vi "Pfeiffer-RVC300.close interface.vi"(0 "i ref in":refnum<vi>, 3 "ms timeout (10000)":i32=10000, 5 "error in (no error)":errorcluster) -> (14 "i ref out":refnum<vi>, 17 "timed out":bool, 19 "error out":errorcluster)   [LabVIEW 2014, in "Pfeiffer-RVC300.lvlib"]
doc: "Closes the interface to the instrument.\n\nLicense Agreement for this software:\n\nCopyright (C)\nMax-Planck-Institut für Kernphysik\nSaupfercheckweg 1\n69117 Heidelberg\nGermany\n\nContact: christopher.borgmann@mpi-hd.mpg.de\n\nThis program is free software: you can redistribute it and/or modify \nit under the terms of the GNU General Public License as published by\nthe Free Software Foundation, either version 3 of the License, or\n(at your option) any later version.\n\nThis program is distributed in the hope that it will be useful,\nbut WITHOUT ANY WARRANTY; without even the implied warranty of\nMERCHANTABILITY or FITNESS FOR A PARTICULAR PURPOSE. See the\nGNU General Public License for more details.\n\nYou should have received a copy of the GNU General Public License\nalong with this program. If not, see <http://www.gnu.org/licenses/>.\n\nMax-Planck-Institut für Kernphysik\nSaupfercheckweg 1, 69117 Heidelberg, Germany\nFor all questions and ideas contact: christopher.borgmann@mpi-hd.mpg.de\nLast update: 08.07.2010"
uses:
  Pfeiffer-RVC300.lvlib
  CS_Core/CSApplicationBaseClasses/DeviceBase/DeviceBase.lvlib
  instr.lib/RVC300/RVC 300.lvlib
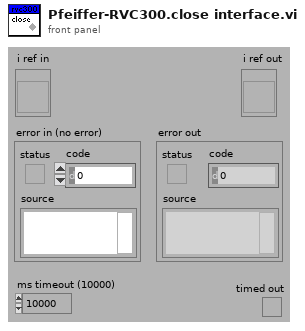
[diagram p1: front panel]
types:
  T1 = typedef "Pfeiffer-RVC300.lvlib/Pfeiffer-RVC300.i attribute.ctl" = cluster{"interfaceInitialized":bool, "VISAResource":refnum<visa-resource-name>, "WaitingTime":u32, "nomValues":T2, "actValues":T2}
  T2 = typedef "Pfeiffer-RVC300.lvlib/Pfeiffer-RVC300.parameters.ctl" = cluster{"regulationMode":T3, "valveType":string, "sensorType":string, "valveState":string, "flow":dbl, "pressure":dbl, "serviceIDs":cluster{"regulationModeID":i32, "valveTypeID":i32, "sensorTypeID":i32, "valveStateID":i32, "flowID":i32, "pressureID":i32}}
  T3 = typedef "Pfeiffer-RVC300.lvlib/Pfeiffer-RVC300.regulation mode.ctl" = enum16{"unknown", "Pressure", "Flow", "Wait"}
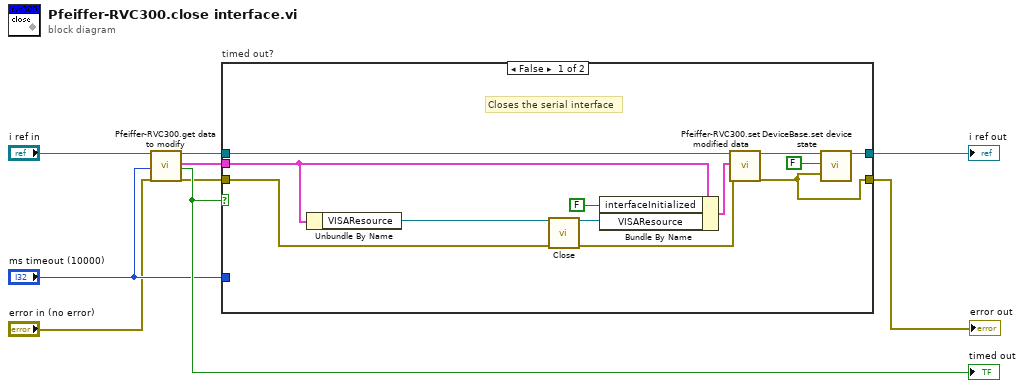
[diagram p0: block diagram]
diagram:
  n1 = call "Pfeiffer-RVC300.get data to modify.vi"("i ref in"="i ref in", "ms timeout (10000)"="ms timeout (10000)", "error in (no error)"="error in (no error)") -> ("i ref out"=w3:refnum<vi>, "i attribute"=w1:T1, "timed out"=w6:bool, "error out"=w2:errorcluster)  [unwired: 13 in]
  "timed out" <- w6
  n2 = case "timed out?" shown="False" w6 {
    tunnel: [w12 w22] -> w8
    tunnel: w3 -> [w18 w22]
    tunnel: [w10 w21] -> w7
    tunnel: w2 -> [w16 w21]
    tunnel: w1 -> [w14 _]
    tunnel: "ms timeout (10000)" -> [_ _]
    frame False {
      # "Closes the serial interface"
      n3 = Unbundle By Name(w14) -> ("VISAResource"=w17:refnum<visa-resource-name>)
      n4 = call "Close.vi"("VISA session"=w17, "error in (no error)"=w16) -> ("error out"=w20:errorcluster)  [unwired: 13 in]
      n5 = Bundle By Name(cluster=w14, "interfaceInitialized"=FALSE, "VISAResource"=w17) -> (w15:T1)
      n6 = call "Pfeiffer-RVC300.set modified data.vi"("i ref in"=w18, "i attribute"=w15, "error in (no error)"=w20) -> ("i ref out"=w13:refnum<vi>, "error out"=w10:errorcluster)  [unwired: 15 in]
      n7 = call "DeviceBase.set device state.vi"("i ref in"=w13, "implicit"=FALSE, "device error"=w10) -> ("i ref out"=w12:refnum<vi>)  [unwired: 14 in, 2 out]
    }
    frame True {
    }
  }
  "error out" <- w7
  "i ref out" <- w8
